vi "SetValue.vi"(8 "error in":errorcluster, 10 "Value":string, 11 "NonNullableString_TruncateAt_255 in":refnum<class "NonNullableString_TruncateAt_255.lvclass">) -> (0 "error out":errorcluster, 3 "NonNullableString_TruncateAt_255 out":refnum<class "NonNullableString_TruncateAt_255.lvclass">)   [LabVIEW 2021, in "ProligentXMLGenerator.lvlib" / "NonNullableString_TruncateAt_255.lvclass"]
uses:
  NonNullableString_TruncateAt_255.lvclass
  NonNullableString_TruncateAt_255.lvclass/NonNullableString_TruncateAt_255.ctl
  NonNullableString/NonNullableString.lvclass
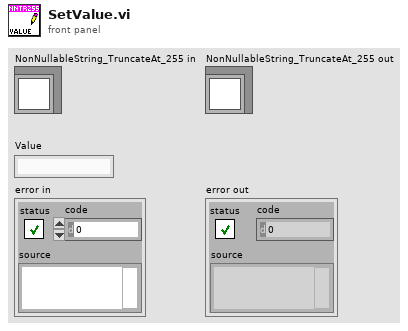
[diagram p1: front panel]
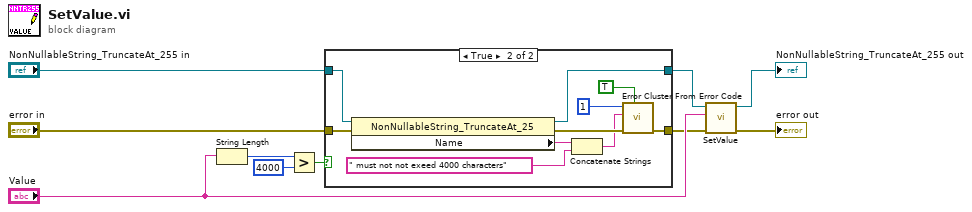
[diagram p0: block diagram]
diagram:
  n1 = String Length(string="Value") -> (length=w5:i32)
  n2 = Greater?(x=w5, y=4000) -> (0:w2:bool)
  n3 = case shown="True" w2 {
    tunnel: "error in" -> [w12 w16]
    tunnel: [w12 w22] -> w3
    tunnel: [w11 w14] -> w1
    tunnel: "NonNullableString_TruncateAt_255 in" -> [w11 w17]
    frame False {
    }
    frame True {
      n4 = property on="Property Node" class="NonNullableString_TruncateAt_25"(reference=w17, error in=w16) -> (reference out=w14:refnum<class "NonNullableString_TruncateAt_255.lvclass">, error out=w15:errorcluster, "Name"=w18:string)
      n5 = Concatenate Strings(w18, " must not not exeed 4000 characters" ("string")) -> (w13:string)
      n6 = call <vilib>:"Error Cluster From Error Code.vi"("show call chain? (False)"=TRUE, "error in (no error)"=w15, "error message (\"\")"=w13, "error code (0)"=1) -> ("error out"=w22:errorcluster)  [unwired: 5 in]
    }
  }
  n7 = call-parent "SetValue.vi"("error in"=w3, "Value"="Value", "String in"=w1) -> ("error out"=→"error out":errorcluster, "String out"=→"NonNullableString_TruncateAt_255 out":refnum<class "NonNullableString_TruncateAt_255.lvclass">)  [unwired: 7 in]
